vi "main.vi"() -> ()   [LabVIEW 2020]
uses:
  <vilib>/Instr/_visa.llb/VISA Configure Serial Port (Instr).vi
panel:
  out "Device name":string
  in  "voltage":dbl(slide) scale=0.0..5.0
  in  "stop":bool
  in  "error in":errorcluster
  out "error out":errorcluster={"status"=FALSE, "code"=1073676294, "source"=""}
  in  "VISA resource name":refnum<visa-resource-name>="COM6"
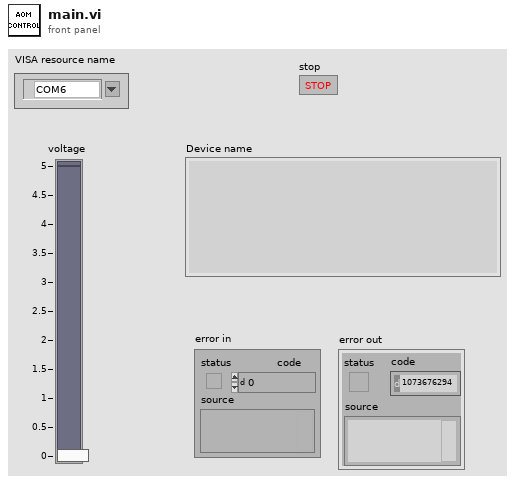
[diagram p1: front panel]
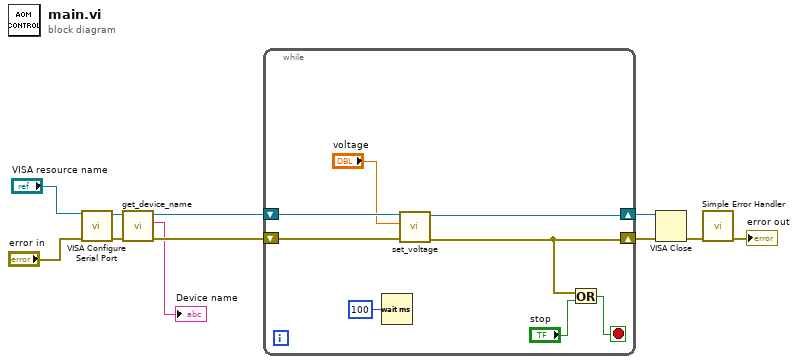
[diagram p0: block diagram]
diagram:
  n1 = call-poly "VISA Configure Serial Port"("VISA resource name"="VISA resource name", "error in (no error)"="error in") -> ("VISA resource name out"=w5:refnum<visa-resource-name>, "error out"=w4:errorcluster)  [unwired: 8 in, 4 out]
  n2 = call "get_device_name.vi"("error in"=w4, "VISA resource name in"=w5) -> ("error out"=w2:errorcluster, "Device name"=→"Device name":string, "VISA resource name out"=w3:refnum<visa-resource-name>)  [unwired: 7 in]
  n3 = while {
    shift-right: [w16] -> w7
    shift-left: w3 -> [w18]
    shift-right: [w15] -> w6
    shift-left: w2 -> [w17]
    stop <- w13 stop-if-true
    n4 = Wait (ms)(milliseconds to wait=u32 100) -> ()  [unwired: 1 out]
    n5 = call "set_voltage.vi"("error in"=w17, "voltage"="voltage", "VISA resource name"=w18) -> ("error out"=w15:errorcluster, "VISA resource name out"=w16:refnum<visa-resource-name>)  [unwired: 6 in, 1 out]
    n6 = Or(x=w15, y="stop") -> (x .or. y?=w13:bool)
  }
  n7 = VISA Close(VISA resource name=w7, error in (no error)=w6) -> (error out=w10:errorcluster)
  n8 = call <vilib>:"Simple Error Handler.vi"("error in (no error)"=w10) -> ("error out"=→"error out":errorcluster)  [unwired: 1 in, 7 out]
